vi "g_HCCRegisterConfig.vi"() -> ()   [LabVIEW 2014]
panel:
  out "Table":string[][](table)=[["HCC Register", "Address", "Value", "Default Values"], ["HCC_REG_0", " 0x00", "", " 0x040402C5"], ["HCC_REG_1", " 0x01", "", " 0xE2810040"], ["HCC_REG_2", " 0x02", "", " 0x00000840"], ["HCC_REG_3", " 0x03", "", " 0x000FFC00"], ["HCC_REG_4", " 0x04", "", " 0x3FF003FF"], ["HCC_REG_5", " 0x05", "", " 0x000FFC00"], ["HCC_REG_6", " 0x06", "", " 0x3FF003FF"], ["HCC_REG_7", " 0x07", "", " 0x000FFC00"], ["HCC_REG_8", " 0x08", "", " 0x00000000"], ["HCC_REG_9", " 0x09", "", " 0x08421094"], ["HCC_REG_10", " 0x10", "", " 0x00111104"], ["HCC_REG_11", " 0x11", "", " 0x01010401"], ["HCC_REG_12", " 0x12", "", " 0x00000000"], ["HCC_REG_13", " 0x13", "", " 0x00700000"], ["HCC_REG_14", " 0x14", "", " 0xFFF00000"], ["HCC_REG_15", " 0x15", "", " 0xFFFFFFFF"], ["HCC_REG_16", " 0x16", "", " 0x00000000"], ["HCC_REG_17", " 0x17", "", " 0x00000000"]]
  in  "Default":bool
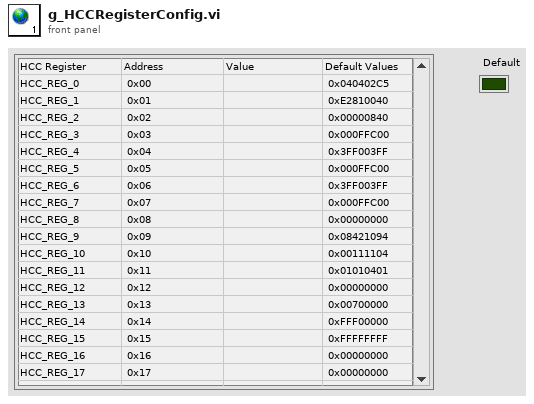
[diagram p1: front panel]
diagram:
